vi "Save-Recall Calibration.vi"(0 "VISA resource name":refnum<visa-resource-name>, 1 "saver's name":string, 2 "saved cal title":string, 5 "save/recall (f : recall)":bool, 7 "file name (read description)":path, 11 "error in (no error)":errorcluster, 12 "saved cal comments":string) -> (3 "recaller's name":string, 4 "VISA resource name out":refnum<visa-resource-name>, 6 "recalled cal comments":string, 8 "recalled cal date":string, 10 "recalled cal time":string, 14 "recalled cal title":string, 15 "error out":errorcluster)   [LabVIEW 2018, in "Agilent 87XX Series.lvlib"]
doc: "This VI for the HP8753B Network Analyzer is used for saving and recalling calibration kits. The number of correction arrays varies from 1 to 12 depending upon the type of correction. Rather than saving each array in a seperate file, this VI combines all the arrays for a calibration into one file. The data is saved in form 1 to conserve disk space. I initially tried to save it in form 2 to keep it small and also allow it to be decoded by those crazy enough to want to do so. For some strange reason, this would not always work with larger numbers of points. Form 3 did work, but it required too much disk space. \n\nNOTE : One path 2-port calibrations include 12 arrays, but the last 6 duplicate the first 6. This VI saves all twelve for simplicity."
uses:
  Agilent 87XX Series.lvlib
panel:
  # "save to file\nrecall from file"
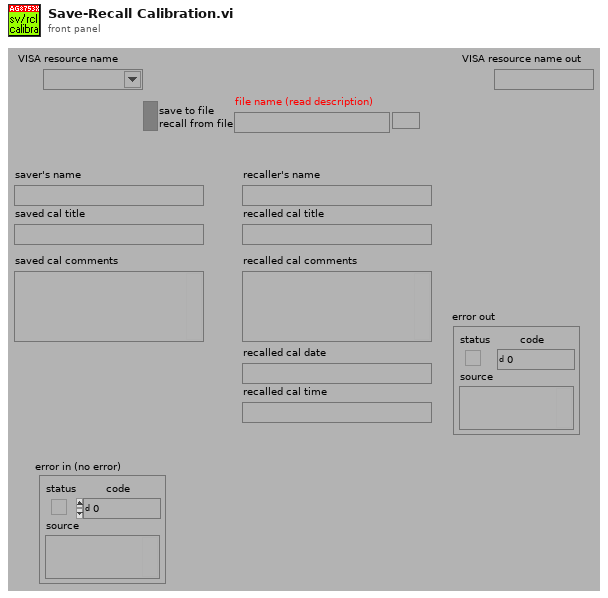
[diagram p1: front panel]
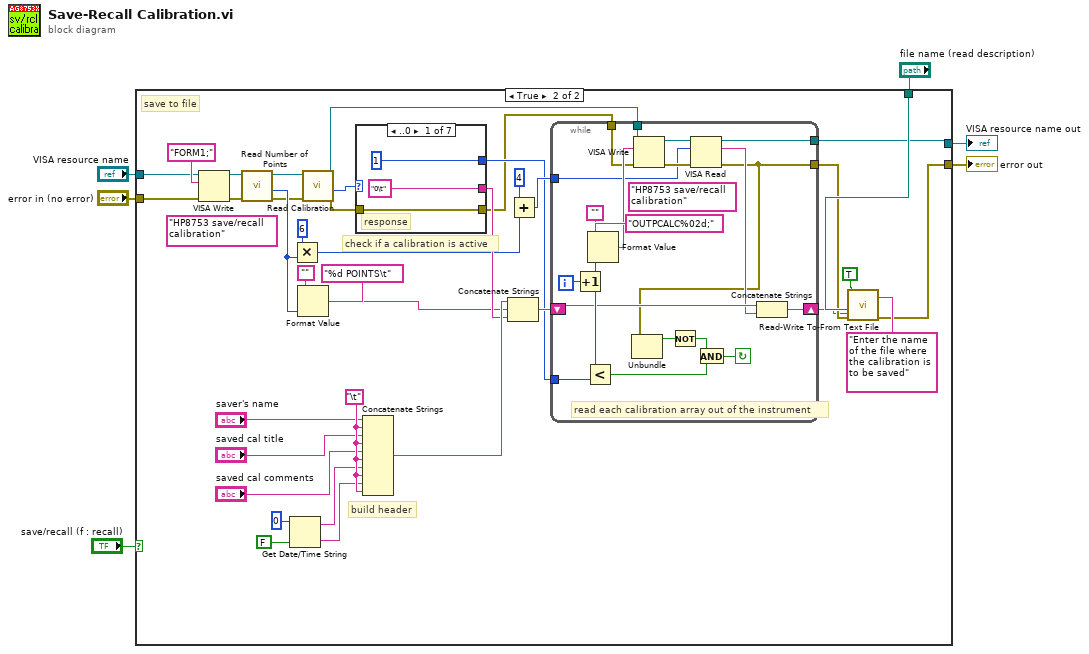
[diagram p0: block diagram]
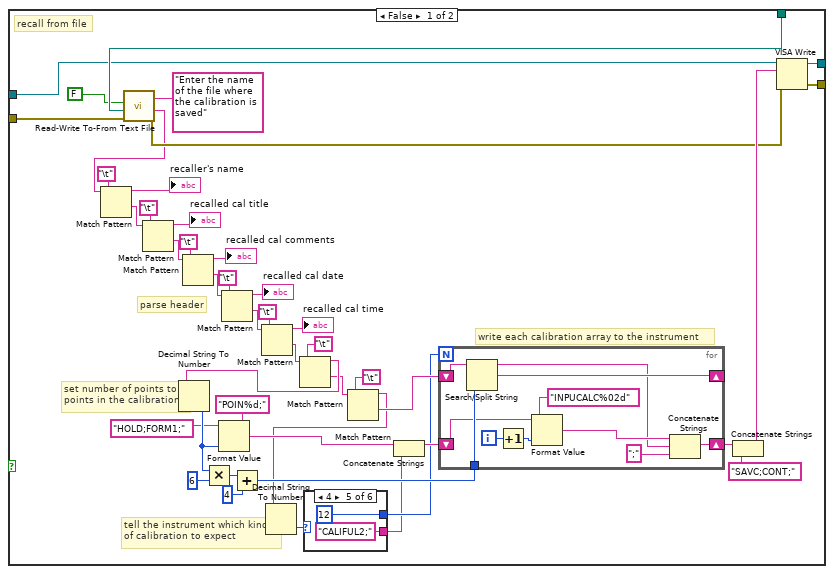
[diagram p2: hidden frame]
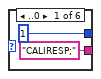
[diagram p3: hidden frame]
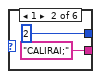
[diagram p4: hidden frame]
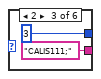
[diagram p5: hidden frame]
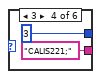
[diagram p6: hidden frame]
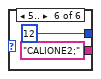
[diagram p7: hidden frame]
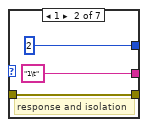
[diagram p8: hidden frame]
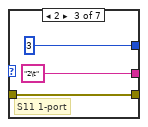
[diagram p9: hidden frame]
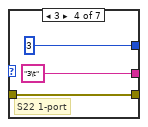
[diagram p10: hidden frame]
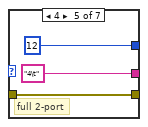
[diagram p11: hidden frame]
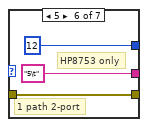
[diagram p12: hidden frame]
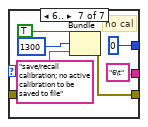
[diagram p13: hidden frame]
diagram:
  n1 = case shown="True" "save/recall (f : recall)" {
    tunnel: "file name (read description)" -> [w25 w101]
    tunnel: "VISA resource name" -> [w10 w81]
    tunnel: "error in (no error)" -> [w12 w80]
    tunnel: [w9 w77] -> w2
    tunnel: [w8 w76] -> w1
    frame False {
      # "write each calibration array to the instrument"
      # "tell the instrument which kind\nof calibration to expect"
      # "set number of points to \npoints in the calibration"
      # "parse header"
      # "recall from file"
      n2 = call "Read-Write To-From Text File.vi"("dialog box prompt"="Enter the name of the file where the calibration is saved", "error in (no error)"=w12, "file name (read description)"=w25, "read/write (f:read)"=FALSE) -> ("error out"=w11:errorcluster, "string which was read"=w7:string)  [unwired: 6 in]
      n3 = Match Pattern(string=w7, regular expression="\t") -> (before substring=→"recaller's name":string, after substring=w48:string)  [unwired: 1 in, 2 out]
      n4 = Match Pattern(string=w48, regular expression="\t") -> (before substring=→"recalled cal title":string, after substring=w47:string)  [unwired: 1 in, 2 out]
      n5 = Match Pattern(string=w47, regular expression="\t") -> (before substring=→"recalled cal comments":string, after substring=w43:string)  [unwired: 1 in, 2 out]
      n6 = Match Pattern(string=w43, regular expression="\t") -> (before substring=→"recalled cal date":string, after substring=w46:string)  [unwired: 1 in, 2 out]
      n7 = Match Pattern(string=w46, regular expression="\t") -> (before substring=→"recalled cal time":string, after substring=w33:string)  [unwired: 1 in, 2 out]
      n8 = Match Pattern(string=w33, regular expression="\t") -> (before substring=w26:string, after substring=w22:string)  [unwired: 1 in, 2 out]
      n9 = Decimal String To Number(string=w26) -> (number=w31:i32)  [unwired: 2 in, 1 out]
      n10 = Multiply(x=w31, y=6) -> (x*y=w29:i32)
      n11 = Format Value(string ("")="HOLD;FORM1;", format string="POIN%d;", value (0)=w31) -> (output string=w19:string)
      n12 = Add(x=w29, y=4) -> (x+y=w27:i32)
      n13 = Match Pattern(string=w22, regular expression="\t") -> (before substring=w17:string, after substring=w21:string)  [unwired: 1 in, 2 out]
      n14 = Decimal String To Number(string=w17) -> (number=w16:i32)  [unwired: 2 in, 1 out]
      n15 = case shown="4" w16 {
        tunnel: [1 2 3 3 12 12] -> w15
        tunnel: ["CALIRESP;" "CALIRAI;" "CALIS111;" "CALIS221;" "CALIFUL2;" "CALIONE2;"] -> w14
        frame ..0 {
        }
        frame 1 {
        }
        frame 2 {
        }
        frame 3 {
        }
        frame 4 {
        }
        frame 5.. {
        }
      }
      n16 = Concatenate Strings(w19, w14) -> (w18:string)
      n17 = for {
        N: w15 -> [_]
        shift-right: [w65] -> w37
        shift-left: w18 -> [w69]
        tunnel: w27 -> [w73]
        shift-right: [w67] -> _
        shift-left: w21 -> [w74]
        i -> [w71]
        n18 = Search/Split String(string=w74, offset (0)=w73) -> (substring before match=w66:string, match + rest of string=w67:string)  [unwired: 1 in, 1 out]
        n19 = Increment(x=w71) -> (x+1=w70:i32)
        n20 = Format Value(string ("")=w69, format string="INPUCALC%02d", value (0)=w70) -> (output string=w68:string)
        n21 = Concatenate Strings(w68, w66, ";") -> (w65:string)
      }
      n22 = Concatenate Strings(w37, "SAVC;CONT;") -> (w35:string)
      n23 = VISA Write(VISA resource name=w10, write buffer=w35, error in (no error)=w11) -> (VISA resource name out=w9:refnum<visa-resource-name>, error out=w8:errorcluster)  [unwired: 1 out]
    }
    frame True {
      (unwired) "HP8753 save/recall calibration"
      w112 = "\t"
      # "build header"
      # "check if a calibration is active"
      # "save to file"
      n24 = VISA Write(VISA resource name=w81, write buffer="FORM1;", error in (no error)=w80) -> (VISA resource name out=w89:refnum<visa-resource-name>, error out=w88:errorcluster)  [unwired: 1 out]
      n25 = call "Read Number of Points.vi"("error in (no error)"=w88, "VISA resource name"=w89) -> ("error out"=w91:errorcluster, "num points"=w94:i32, "VISA resource name out"=w98:refnum<visa-resource-name>)  [unwired: 7 in]
      n26 = Get Date/Time String(date format (0)=0, want seconds? (F)=FALSE) -> (date string=w110:string, time string=w111:string)  [unwired: 1 in]
      n27 = Multiply(x=6, y=w94) -> (x*y=w92:i32)
      n28 = Format Value(string ("")="", format string="%d POINTS\t", value (0)=w94) -> (output string=w93:string)
      n29 = call "Read Calibration.vi"("error in (no error)"=w91, "VISA resource name"=w98) -> ("error out"=w79:errorcluster, "cal type"=w90:i32, "VISA resource name out"=w83:refnum<visa-resource-name>)  [unwired: 7 in]
      n30 = case shown="..0" w90 {
        tunnel: [1 2 3 3 12 12 0] -> w84
        tunnel: ["0\t" "1\t" "2\t" "3\t" "4\t" "5\t" "6\t"] -> w99
        tunnel: w79 -> [w133 w136 w139 w142 w145 w148 _]
        tunnel: [w133 w136 w139 w142 w145 w148 w152] -> w78
        frame ..0 {
          # "response"
        }
        frame 1 {
          # "response and isolation"
        }
        frame 2 {
          # "S11 1-port"
        }
        frame 3 {
          # "S22 1-port"
        }
        frame 4 {
          # "full 2-port"
        }
        frame 5 {
          # "HP8753 only"
          # "1 path 2-port"
        }
        frame 6.. {
          # "no cal"
          n31 = Bundle(TRUE, 1300, "save/recall calibration; no active calibration to be saved to file") -> (w152:errorcluster)  [unwired: 1 in]
        }
      }
      n32 = Concatenate Strings("saver's name", w112, "saved cal title", w112, "saved cal comments", w112, w110, w112, w111, w112) -> (w104:string)
      n33 = Concatenate Strings(w104, w93, w99) -> (w85:string)
      n34 = Add(x=4, y=w92) -> (x+y=w86:i32)
      n35 = while {
        tunnel: [w115] -> w82
        tunnel: [w116] -> w77
        tunnel: w78 -> [w117]
        tunnel: w83 -> [w118]
        tunnel: w84 -> [w124]
        tunnel: w86 -> [w114]
        shift-left: w85 -> [w126]
        shift-right: [w127] -> w75
        i -> [w123]
        stop <- w119 continue-if-true
        (unwired) "HP8753 save/recall calibration"
        # "read each calibration array out of the instrument"
        n36 = Increment(x=w123) -> (x+1=w128:i32)
        n37 = Less?(x=w128, y=w124) -> (x < y?=w120:bool)
        n38 = Format Value(string ("")="", format string="OUTPCALC%02d;", value (0)=w128) -> (output string=w129:string)
        n39 = VISA Write(VISA resource name=w118, write buffer=w129, error in (no error)=w117) -> (VISA resource name out=w113:refnum<visa-resource-name>, error out=w132:errorcluster)  [unwired: 1 out]
        n40 = VISA Read(VISA resource name=w113, byte count=w114, error in (no error)=w132) -> (VISA resource name out=w116:refnum<visa-resource-name>, read buffer=w125:string, error out=w115:errorcluster)  [unwired: 1 out]
        n41 = Unbundle(w115) -> ("status"=w122:bool)  [unwired: 2 out]
        n42 = Not(x=w122) -> (.not. x?=w121:bool)
        n43 = And(x=w121, y=w120) -> (x .and. y?=w119:bool)
        n44 = Concatenate Strings(w126, w125) -> (w127:string)
      }
      n45 = call "Read-Write To-From Text File.vi"("string to be written"=w75, "dialog box prompt"="Enter the name of the file where the calibration is to be saved", "error in (no error)"=w82, "file name (read description)"=w101, "read/write (f:read)"=TRUE) -> ("error out"=w76:errorcluster)  [unwired: 5 in, 1 out]
    }
  }
  "error out" <- w1
  "VISA resource name out" <- w2
